vi "Error Query.vi"(8 "error in (no error)":errorcluster, 11 "VISA resource name":refnum<visa-resource-name>) -> (0 "error out":errorcluster, 1 "Error Message":string, 2 "Error Code":i32[](array[numeric]), 3 "VISA resource name out":refnum<visa-resource-name>)   [LabVIEW 2018, in "SF-10.lvlib"]
doc: "Queries the instrument for any errors in the instrument's error queue. It will continue to read errors until all errors have been read from the instrument. Any errors will be returned in the <B>error out</B> control.\n\n<B>Note:</B>\nThis VI is called automatically by most driver VIs so it is not usually necessary to call this in an application."
uses:
  <instrlib>/SF-10/SF-10.lvlib
panel:
  # "EDIT: Note: The Error Query VI is included as a subVI in all driver VIs except low-level API VIs. If the instrument does not support error query, then remove the VI and remove subVI calls in each instrument driver VI that calls it."
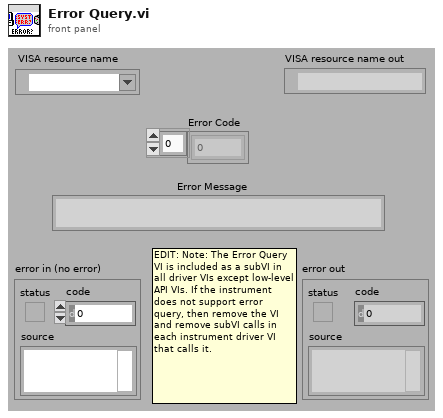
[diagram p1: front panel]
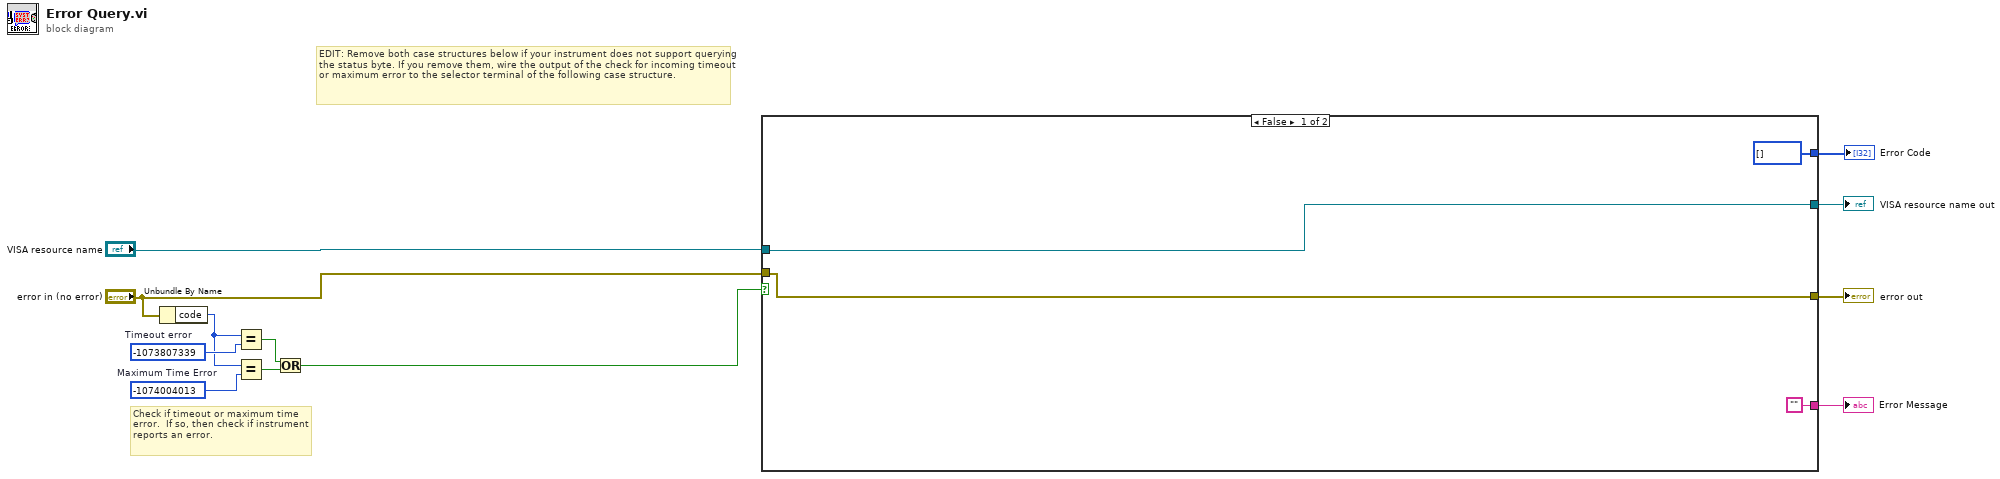
[diagram p0: block diagram]
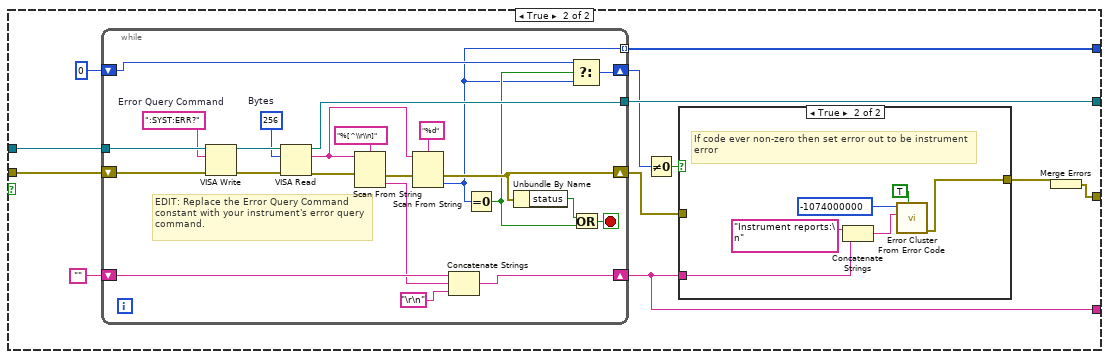
[diagram p2: hidden frame]
diagram:
  w6 = -1074004013  # Maximum Time Error
  w8 = -1073807339  # Timeout error
  # "Check if timeout or maximum time error.  If so, then check if instrument reports an error."
  # "EDIT: Remove both case structures below if your instrument does not support querying the status byte. If you remove them, wire the output of the check for incoming timeout or maximum error to the selector terminal of the following case structure."
  n1 = Unbundle By Name("error in (no error)") -> ("code"=w7:i32)
  n2 = Equal?(x=w7, y=w8) -> (x = y?=w4:bool)
  n3 = Equal?(x=w7, y=w6) -> (x = y?=w5:bool)
  n4 = Or(x=w4, y=w5) -> (x .or. y?=w2:bool)
  n5 = case shown="False" w2 {
    tunnel: [w16 w28] -> w12
    tunnel: "VISA resource name" -> [w16 w27]
    tunnel: [w13 w25] -> w11
    tunnel: ["" w20] -> w10
    tunnel: [i32[] [] w19] -> w9
    tunnel: "error in (no error)" -> [w13 w17]
    frame False {
    }
    frame True {
      n6 = while {
        tunnel: [w58] -> w28
        tunnel: w27 -> [w57]
        shift-right: [w45] -> w20
        shift-left: "" -> [w48]
        shift-right: [w43] -> w21
        shift-left: 0 -> [w44]
        shift-right: [w41] -> w18
        shift-left: w17 -> [w42]
        tunnel: [w36] -> w19 mode=indexing
        stop <- w51 stop-if-true
        w55 = u32 256  # Bytes
        w53 = ":SYST:ERR?"  # Error Query Command
        # "EDIT: Replace the Error Query Command constant with your instrument's error query command."
        n7 = VISA Write(VISA resource name=w57, write buffer=w53, error in (no error)=w42) -> (VISA resource name out=w56:refnum<visa-resource-name>, error out=w54:errorcluster)  [unwired: 1 out]
        n8 = VISA Read(VISA resource name=w56, byte count=w55, error in (no error)=w54) -> (VISA resource name out=w58:refnum<visa-resource-name>, read buffer=w49:string, error out=w40:errorcluster)  [unwired: 1 out]
        n9 = Scan From String(format string="%[^\\r\\n]", input string=w49, error in=w40) -> (error out=w39:errorcluster, output 1=w46:string)  [unwired: 2 in, 2 out]
        n10 = Scan From String(format string="%d", input string=w49, error in=w39) -> (error out=w41:errorcluster, output 1=w36:i32)  [unwired: 2 in, 2 out]
        n11 = Concatenate Strings(w48, w46, "\r\n") -> (w45:string)
        n12 = Equal To 0?(x=w36) -> (x = 0?=w37:bool)
        n13 = Unbundle By Name(w41) -> ("status"=w38:bool)
        n14 = Select(t=w44, s=w37, f=w36) -> (s? t:f=w43:i32)
        n15 = Or(x=w38, y=w37) -> (x .or. y?=w51:bool)
      }
      n16 = Not Equal To 0?(x=w21) -> (x != 0?=w23:bool)
      n17 = case shown="True" w23 {
        tunnel: w20 -> [_ w34]
        tunnel: [w29 w30] -> w22
        tunnel: w18 -> [w29 _]
        frame False {
        }
        frame True {
          # "If code ever non-zero then set error out to be instrument error"
          n18 = Concatenate Strings("Instrument reports:\n" ("Source"), w34) -> (w31:string)
          n19 = call <vilib>:"Error Cluster From Error Code.vi"("show call chain? (False)"=TRUE, "error message (\"\")"=w31, "error code (0)"=-1074000000 ("Code")) -> ("error out"=w30:errorcluster)  [unwired: 6 in]
        }
      }
      n20 = Merge Errors(w22) -> (w25:errorcluster)
    }
  }
  "VISA resource name out" <- w12
  "error out" <- w11
  "Error Message" <- w10
  "Error Code" <- w9
